vi "Coord Filter.vi"(11 "Coordinates":T1(array[cluster])) -> (1 "Filtered Co-ordinates":T1(array[cluster]))   [LabVIEW 2017]
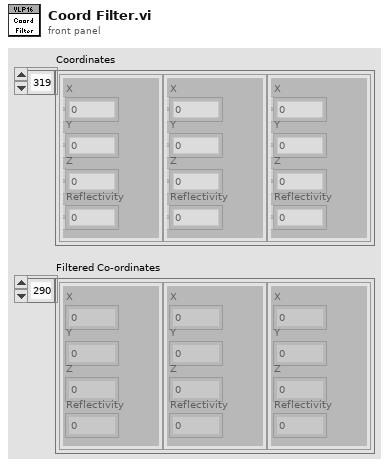
[diagram p1: front panel]
types:
  T1 = cluster{"X":dbl, "Y":dbl, "Z":dbl, "Reflectivity":dbl}[]
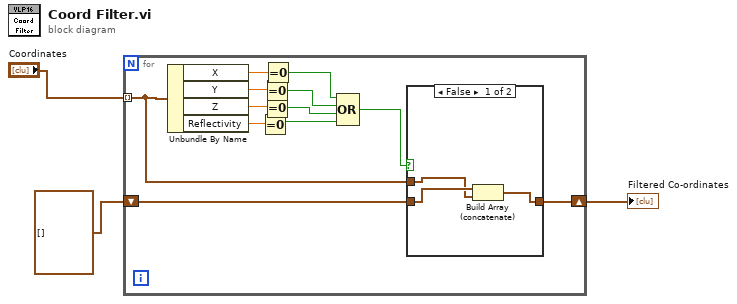
[diagram p0: block diagram]
diagram:
  n1 = for {
    tunnel: "Coordinates" -> [w4] mode=indexing
    shift-right: [w6] -> w1
    shift-left: cluster{dbl, dbl, dbl, dbl}[] [] -> [w7]
    n2 = Unbundle By Name(w4) -> ("X"=w15:dbl, "Y"=w14:dbl, "Z"=w13:dbl, "Reflectivity"=w12:dbl)
    n3 = Equal To 0?(x=w12) -> (x = 0?=w8:bool)
    n4 = Equal To 0?(x=w14) -> (x = 0?=w10:bool)
    n5 = Equal To 0?(x=w13) -> (x = 0?=w9:bool)
    n6 = Equal To 0?(x=w15) -> (x = 0?=w11:bool)
    n7 = Compound Arithmetic op=OR(w11, w10, w9, w8) -> (w5:bool)
    n8 = case shown="False" w5 {
      tunnel: w7 -> [w18 w19]
      tunnel: [w16 w19] -> w6
      tunnel: w4 -> [w17 _]
      frame False {
        n9 = Build Array (concatenate)(w18, w17) -> (w16:T1)
      }
      frame True {
      }
    }
  }
  "Filtered Co-ordinates" <- w1
